vi "MPUSBOpen.vi"(6 "dwReserved":u32, 7 "dwDir":enum16{"Write", "Read"}(ring), 8 "error in (no error)":errorcluster, 9 "pEP":string="\\MCHP_EP1", 10 "pVID_PID":string="vid_04d8&pid_000c", 11 "instance":u32) -> (0 "error out":errorcluster, 2 "HANDLE":u32 format="%04x", 3 "instanceOut":u32)   [LabVIEW 2019]
doc: "// MPUSBOpen : Returns the handle to the endpoint pipe with matching VID & PID\n//\n// All pipes are opened with the FILE_FLAG_OVERLAPPED attribute.\n// This allows MPUSBRead,MPUSBWrite, and MPUSBReadInt to have a time-out value.\n//\n// Note: Time-out value has no meaning for Isochronous pipes.\n\nWritten by: Complete Automated Solutions\nwww.CompleteAutomatedSolutions.com"
uses:
  mpusbapi.dll
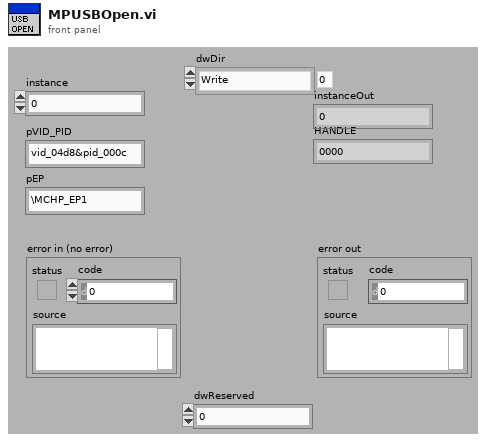
[diagram p1: front panel]
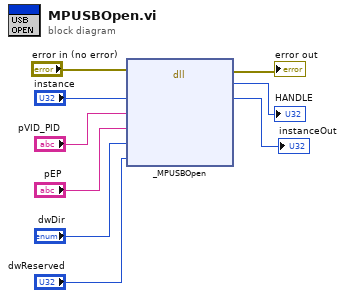
[diagram p0: block diagram]
diagram:
  n1 = dll-call lib="C:/Users/z003r4zd/Desktop/Point Contact Mods 2019/Automation/Actuonix/LAC+Labview+Example/Actuonix_LAC_LabVIEW_Example/USB_VIs/mpusbapi.dll" fn="_MPUSBOpen"(error in="error in (no error)", "instance"="instance", "pVID_PID"="pVID_PID", "pEP"="pEP", "dwDir"="dwDir", "dwReserved"="dwReserved") -> (error out=→"error out":errorcluster, "return_value"=→"HANDLE":u32, "instance"=→"instanceOut":u32)  [unwired: 5 in, 2 out]
